vi "LogMap_FieldOrder.vi"(5 "Set (F)":bool, 8 "Error In":errorcluster, 11 "FieldOrder":string[](array[string])) -> (0 "Error Out":errorcluster, 3 "FieldOrder out":string[](array[string]))   [LabVIEW 2020, in "ORM.lvlib" / "LogMap.lvclass"]
uses:
  LogMap.lvclass
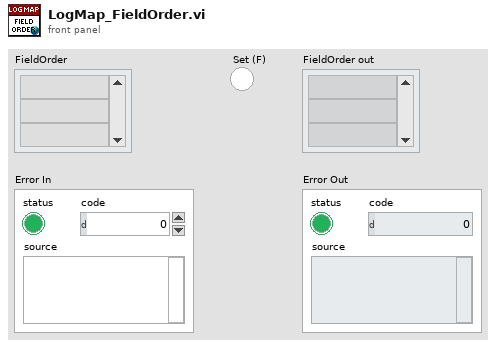
[diagram p1: front panel]
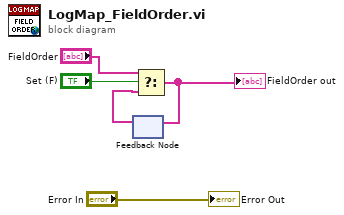
[diagram p0: block diagram]
diagram:
  n1 = feedback #1() -> (w1:string[])  [unwired: 1 in]
  n2 = Select(t="FieldOrder", s="Set (F)", f=w1) -> (s? t:f=w2:string[])
  "FieldOrder out" <- w2
  n3 = feedback-in #1(w2) -> ()
  "Error Out" <- "Error In"
